vi "read_MonitorGain_subVI.vi"(5 "Num Bytes to Fetch (64) in":u8=64 min=1, 6 "Aardvark Handle in":i32 min=0, 8 "error in (no error)":errorcluster, 9 "Address (0x50) in":u16=80 max=1023 format="%.0x") -> (3 "Gain":dbl)   [LabVIEW 2014]
uses:
  aardvark.dll
panel:
  out "error out":errorcluster
  in  "Aardvark Handle":i32 min=0
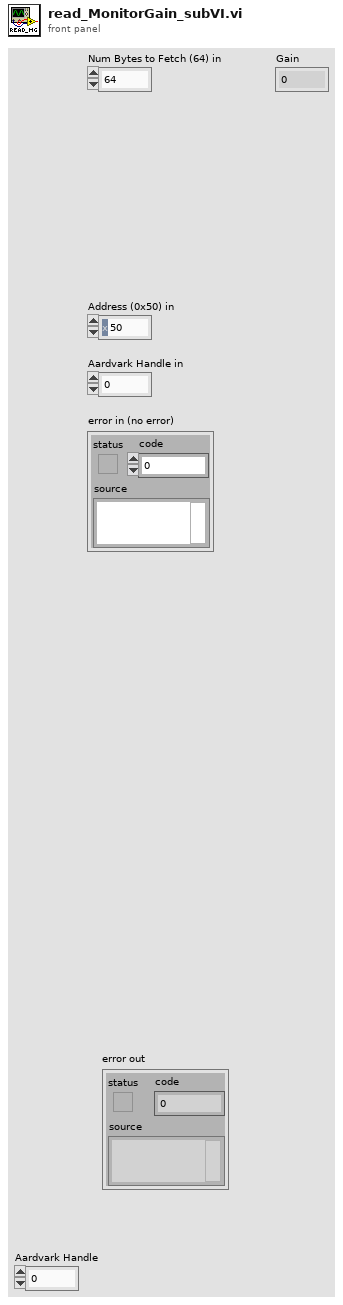
[diagram p1: front panel]
types:
  T1 = cluster{"Boolean array[0]":bool, "Boolean array[1]":bool, "Boolean array[2]":bool, "Boolean array[3]":bool, "Boolean array[4]":bool, "Boolean array[5]":bool, "Boolean array[6]":bool, "Boolean array[7]":bool, "Boolean array[8]":bool}
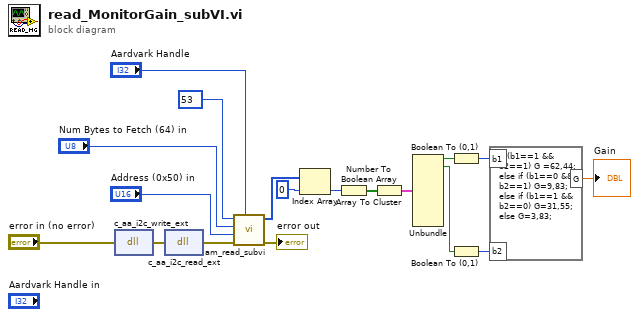
[diagram p0: block diagram]
diagram:
  n1 = dll-call lib="C:/Users/p282652/Documents/LabVIEW Data/Demonstrator/labviewFunctions_AM/aardvark.dll" fn="c_aa_i2c_write_ext"(error in="error in (no error)") -> (error out=w18:errorcluster)  [unwired: 3 in, 1 out]
  n2 = dll-call lib="C:/Users/p282652/Documents/LabVIEW Data/Demonstrator/labviewFunctions_AM/aardvark.dll" fn="c_aa_i2c_read_ext"(error in=w18) -> (error out=w4:errorcluster)  [unwired: 3 in, 1 out]
  n3 = call "am_read_subvi.vi"("Aardvark Handle in"="Aardvark Handle", "error in (no error)"=w4, "Address (0x50) in"="Address (0x50) in", "Num Bytes to Fetch (64)"="Num Bytes to Fetch (64) in", "Memory ADD"=u16 53) -> ("error out"=→"error out":errorcluster, "Array"=w2:u8[])  [unwired: 5 in]
  n4 = Index Array(array=w2, index=0) -> (element=w13:u8)
  n5 = Number To Boolean Array(number=w13) -> (Boolean array=w12:bool[])
  n6 = Array To Cluster(array=w12) -> (cluster=w15:T1)
  n7 = Unbundle(w15) -> ("Boolean array[0]"=w11:bool, "Boolean array[1]"=w9:bool)  [unwired: 7 out]
  n8 = Boolean To (0,1)(Boolean=w11) -> (0, 1=w10:i16)
  n9 = Boolean To (0,1)(Boolean=w9) -> (0, 1=w8:i16)
  n10 = formula code="if (b1==1 && b2==1) G =62,44; else if (b1==0 && b2==1) G=9,83; else if (b1==1 && b2==0) G=31,55; else G=3,83;"("b1"=w10, "b2"=w8) -> ("G"=→"Gain":dbl)
